vi "Is Tail Hit.vi"(8 "error in (no error)":errorcluster, 11 "Snake in":refnum<class "Snake.lvclass">) -> (0 "error out":errorcluster, 2 "Tail Hit!?":bool, 3 "Snake out":refnum<class "Snake.lvclass">)   [LabVIEW 2015, in "Snake.lvclass"]
uses:
  Snake.lvclass
  Snake.lvclass/Snake.ctl
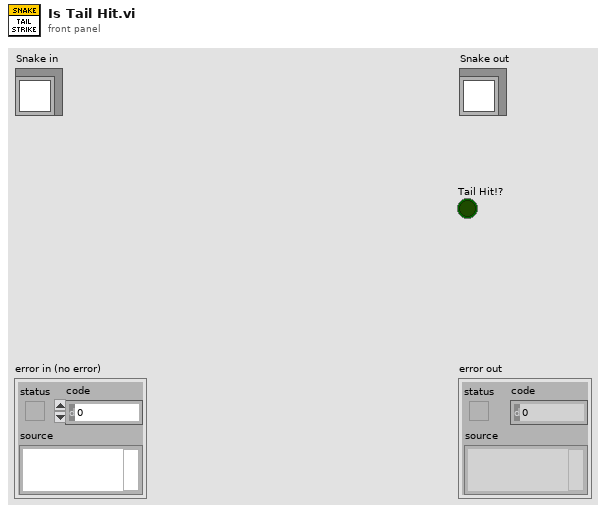
[diagram p1: front panel]
types:
  T1 = typedef "Coordinates.ctl" = cluster{"X":i32, "Y":i32}
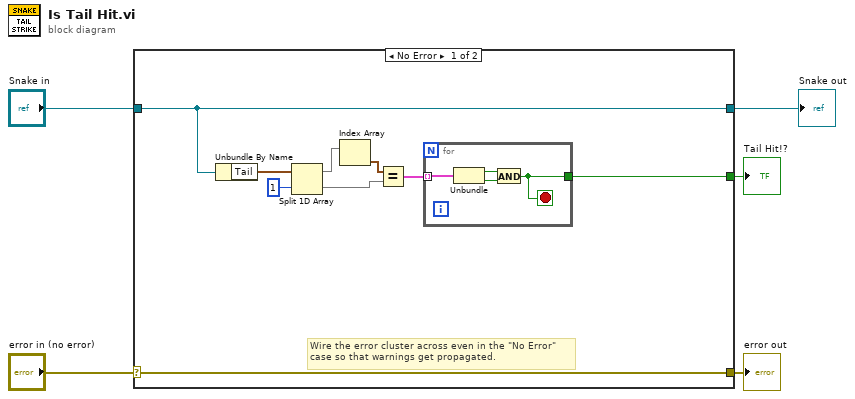
[diagram p0: block diagram]
diagram:
  n1 = case shown="No Error" "error in (no error)" {
    selector: "error in (no error)" -> [w14 w20]
    tunnel: [w14 w20] -> w4
    tunnel: [w13 w19] -> w2
    tunnel: "Snake in" -> [w13 w19]
    tunnel: [w11 _] -> w1
    frame No Error {
      # "Wire the error cluster across even in the \"No Error\"\ncase so that warnings get propagated."
      n2 = Unbundle By Name(w13) -> ("Tail"=w8:T1[])
      n3 = Split 1D Array(array=w8, index=1) -> (first subarray=w7:T1[], second subarray=w10:T1[])
      n4 = Index Array(array=w7) -> (element=w6:T1)  [unwired: 1 in]
      n5 = Equal?(x=w6, y=w10) -> (x = y?=w12:cluster{"X":bool, "Y":bool}[])
      n6 = for {
        tunnel: w12 -> [w18] mode=indexing
        tunnel: [w15] -> w11
        stop <- w15 stop-if-true
        n7 = Unbundle(w18) -> ("X"=w17:bool, "Y"=w16:bool)
        n8 = And(x=w17, y=w16) -> (x .and. y?=w15:bool)
      }
    }
    frame Error {
    }
  }
  "error out" <- w4
  "Snake out" <- w2
  "Tail Hit!?" <- w1
